vi "Untitled 2 (SubVI).vi"(10 "Array":string[](array[string]), 11 "String in":string) -> (3 "String out":string)   [LabVIEW 2015]
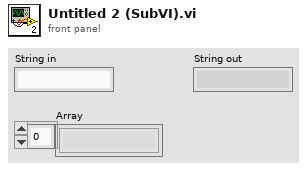
[diagram p1: front panel]
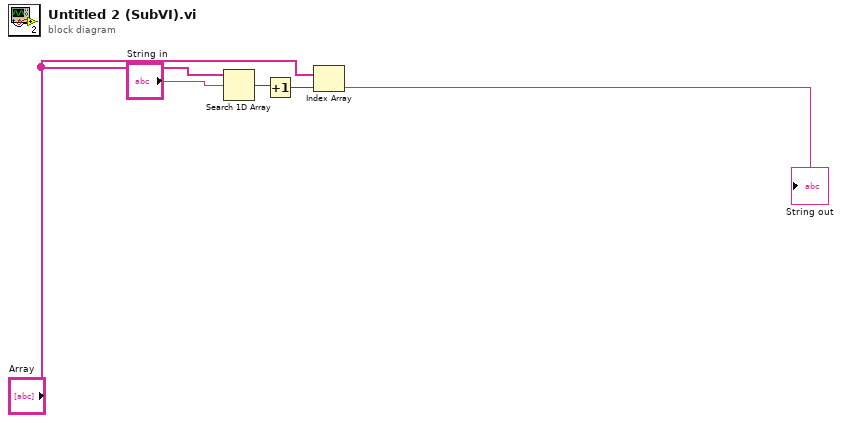
[diagram p0: block diagram]
diagram:
  n1 = Search 1D Array(1D array="Array", element="String in") -> (index of element=w2:i32)  [unwired: 1 in]
  n2 = Increment(x=w2) -> (x+1=w1:i32)
  n3 = Index Array(array="Array", index=w1) -> (element=→"String out":string)
